vi "test-unscented-kalman-filter-0.vi"() -> (3 "All Tests Good":bool)   [LabVIEW 2019]
uses:
  <vilib>/Rock Robotics/WPI/ThirdParty/JAS_Junk/TrajLib/UNSCENTED_KALMAN_FILTER.ctl
  <vilib>/Analysis/Matrix/Datatypes/RealMatrix.ctl
  <vilib>/Rock Robotics/WPI/ThirdParty/JAS_Junk/TrajLib/MERWE_SCALED_SIGMA_PTS.ctl
  <vilib>/Rock Robotics/WPI/ThirdParty/JAS_Junk/TrajLib/CALLBACK_FUNC_TYPE.ctl
  <vilib>/Rock Robotics/WPI/ThirdParty/JAS_Junk/TrajLib/Rotation2d_CreateAngle.vi
  <vilib>/Rock Robotics/WPI/ThirdParty/JAS_Junk/TrajLib/Translation2d_Create.vi
  <vilib>/Rock Robotics/WPI/ThirdParty/JAS_Junk/TrajLib/Trajectory_Library.lvlib
  <vilib>/Analysis/Matrix/NI_Matrix.lvlib
panel:
  out "Error 7":bool
  out "JacobU":T1
  out "Y 2":T1
  out "out UnscentedKalmanFiilter 6":T2
  out "Error 6":bool
  out "out UnscentedKalmanFiilter 5":T2
  out "Error 5":bool
  out "out UnscentedKalmanFiilter 4":T2
  out "Error 4":errorcluster
  out "UnscentedKalmanFiilter 2":T2
  out "Y":T1
  out "out UnscentedKalmanFiilter 3":T2
  out "Error 3":bool
  out "out UnscentedKalmanFiilter 2":T2
  out "Error 2":bool
  out "out UnscentedKalmanFiilter":T2
  out "Error":errorcluster
  out "UnscentedKalmanFiilter":T2
  # "State Estimate <Statess,1>"
  # "<States, States>"
  # "<States, ?>"
  # "<Statess,  States>"
  # "<Outputs, Outputs>"
  # "<?, 1>"
  # "<?, 1>"
  # "State Estimate <Statess,1>"
  # "<States, States>"
  # "<States, ?>"
  # "<Statess,  States>"
  # "<Outputs, Outputs>"
  # "<?, 1>"
  # "<?, 1>"
  # "State Estimate <Statess,1>"
  # "<States, States>"
  # "<States, ?>"
  # "<Statess,  States>"
  # "<Outputs, Outputs>"
  # "<?, 1>"
  # "<?, 1>"
  # "State Estimate <Statess,1>"
  # "<States, States>"
  # "<States, ?>"
  # "<Statess,  States>"
  # "<Outputs, Outputs>"
  # "<?, 1>"
  # "<?, 1>"
  # "State Estimate <Statess,1>"
  # "<States, States>"
  # "<States, ?>"
  # "<Statess,  States>"
  # "<Outputs, Outputs>"
  # "<?, 1>"
  # "<?, 1>"
  # "State Estimate <Statess,1>"
  # "<States, States>"
  # "<States, ?>"
  # "<Statess,  States>"
  # "<Outputs, Outputs>"
  # "<?, 1>"
  # "<?, 1>"
  # "State Estimate <Statess,1>"
  # "<States, States>"
  # "<States, ?>"
  # "<Statess,  States>"
  # "<Outputs, Outputs>"
  # "<?, 1>"
  # "<?, 1>"
  # "State Estimate <Statess,1>"
  # "<States, States>"
  # "<States, ?>"
  # "<Statess,  States>"
  # "<Outputs, Outputs>"
  # "<?, 1>"
  # "<?, 1>"
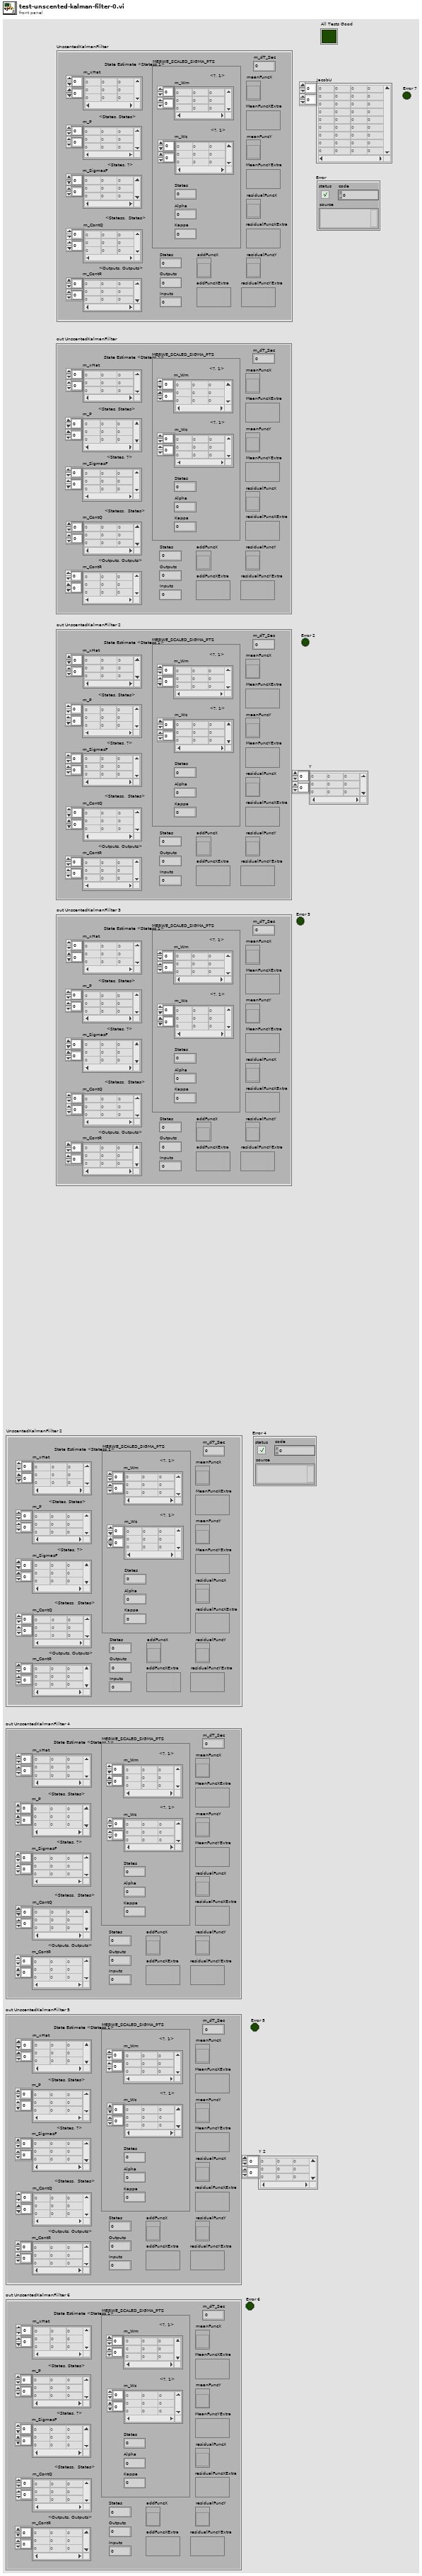
[diagram p1: front panel]
types:
  T1 = typedef "NI_Matrix.lvlib/RealMatrix.ctl" = dbl[][]
  T2 = typedef "Trajectory_Library.lvlib/UNSCENTED_KALMAN_FILTER.ctl" = cluster{"m_P":T1, "m_xHat":T1, "States":i32, "Outputs":i32, "m_ContR":T1, "m_ContQ":T1, "m_SigmasF":T1, "m_dT_Sec":dbl, "MERWE_SCALED_SIGMA_PTS":T3, "meanFuncX":T4, "meanFuncY":T4, "residualFuncX":T4, "residualFuncY":T4, "addFuncX":T4, "addFuncXExtra":variant, "residualFuncYExtra":variant, "residualFuncXExtra":variant, "MeanFuncYExtra":variant, "MeanFuncXExtra":variant, "Inputs":i32}
  T3 = typedef "Trajectory_Library.lvlib/MERWE_SCALED_SIGMA_PTS.ctl" = cluster{"m_Wm":T1, "States":i32, "Alpha":dbl, "m_Wc":T1, "Kappa":i32}
  T4 = typedef "Trajectory_Library.lvlib/CALLBACK_FUNC_TYPE.ctl" = refnum<vi>
  T5 = typedef "Trajectory_Library.lvlib/POSE2D.ctl" = cluster{"TRANSLATION":T6, "ROTATION":T7}
  T6 = typedef "Trajectory_Library.lvlib/TRANSLATION2D.ctl" = cluster{"X":dbl, "Y":dbl}
  T7 = typedef "Trajectory_Library.lvlib/ROTATION2D.ctl" = cluster{"VALUE":dbl, "COS":dbl, "SIN":dbl}
  T8 = typedef "Trajectory_Library.lvlib/TRAJ_CONFIG.ctl" = cluster{"MaxVelocity":dbl, "Max Acceleration":dbl, "StartVelocity":dbl, "End Velocity":dbl, "Reversed":bool, "DiffDrKineConstntDefined":bool, "CentAcellConstntDefined":bool, "DiffDrVoltConstntDefined":bool, "DIFF_DRIVE_KINE_CONSTRAINT":T9, "CENTRIPETAL_ACCEL_CONSTRAINT":T11, "SwerveDrKineConstntDefined":bool, "SWERVE_DRIVE_KINE_CONSTRAINT":T12, "DIFF_DRIVE_VOLTAGE_CONSTRAINT":T14, "MECANUM_DRIVE_KINE_CONSTRAINT":T16, "MecanumDrKineConstntDefined":bool}
  T9 = typedef "Trajectory_Library.lvlib/TRAJ_CONSTRAINT_DIIF_DRIVE_KINEMATICS.ctl" = cluster{"Max Speed (M/S)":dbl, "DIFF_DRIVE_KINEMATICS":T10, "Max Accel (M/S2)":dbl}
  T10 = typedef "Trajectory_Library.lvlib/DIFF_DRIVE_KINEMATICS.ctl" = cluster{"TrackWidth_Meters":dbl}
  T11 = typedef "Trajectory_Library.lvlib/TRAJ_CONSTRAINT_CENTRIPETAL_ACCEL.ctl" = cluster{"Max Cent Accel":dbl}
  T12 = typedef "Trajectory_Library.lvlib/TRAJ_CONSTRAINT_SWERVE_DRIVE_KINEMATICS.ctl" = cluster{"Max Speed (M/S)":dbl, "SwerveKinematics":T13}
  T13 = typedef "Trajectory_Library.lvlib/SWERVE_DRIVE_KINEMATICS.ctl" = cluster{"NumModules":i32, "InverseKinematics":T1, "ForwardKinematics":T1, "Modules":T6[], "PrevCoR":T6}
  T14 = typedef "Trajectory_Library.lvlib/TRAJ_CONSTRAINT_DIIF_DRIVE_VOLTAGE.ctl" = cluster{"Max Voltage":dbl, "DIFF_DRIVE_KINEMATICS":T10, "SIMPLE_MOTOR_FF":T15}
  T15 = typedef "Trajectory_Library.lvlib/SIMPLE_MOTOR_FF.ctl" = cluster{"Ks":dbl, "Kv":dbl, "Ka":dbl}
  T16 = typedef "Trajectory_Library.lvlib/TRAJ_CONSTRAINT_MECA_DRIVE_KINEMATICS.ctl" = cluster{"Max Speed (M/S)":dbl, "MECA_DRIVE_KINEMATICS":T17}
  T17 = typedef "Trajectory_Library.lvlib/MECA_DRIVE_KINEMATICS.ctl" = cluster{"FrontLeft":T6, "FrontRight":T6, "RearLeft":T6, "RearRight":T6, "InverseKinematics":T1, "ForwardKinematics":T1, "PrevCoR":T6}
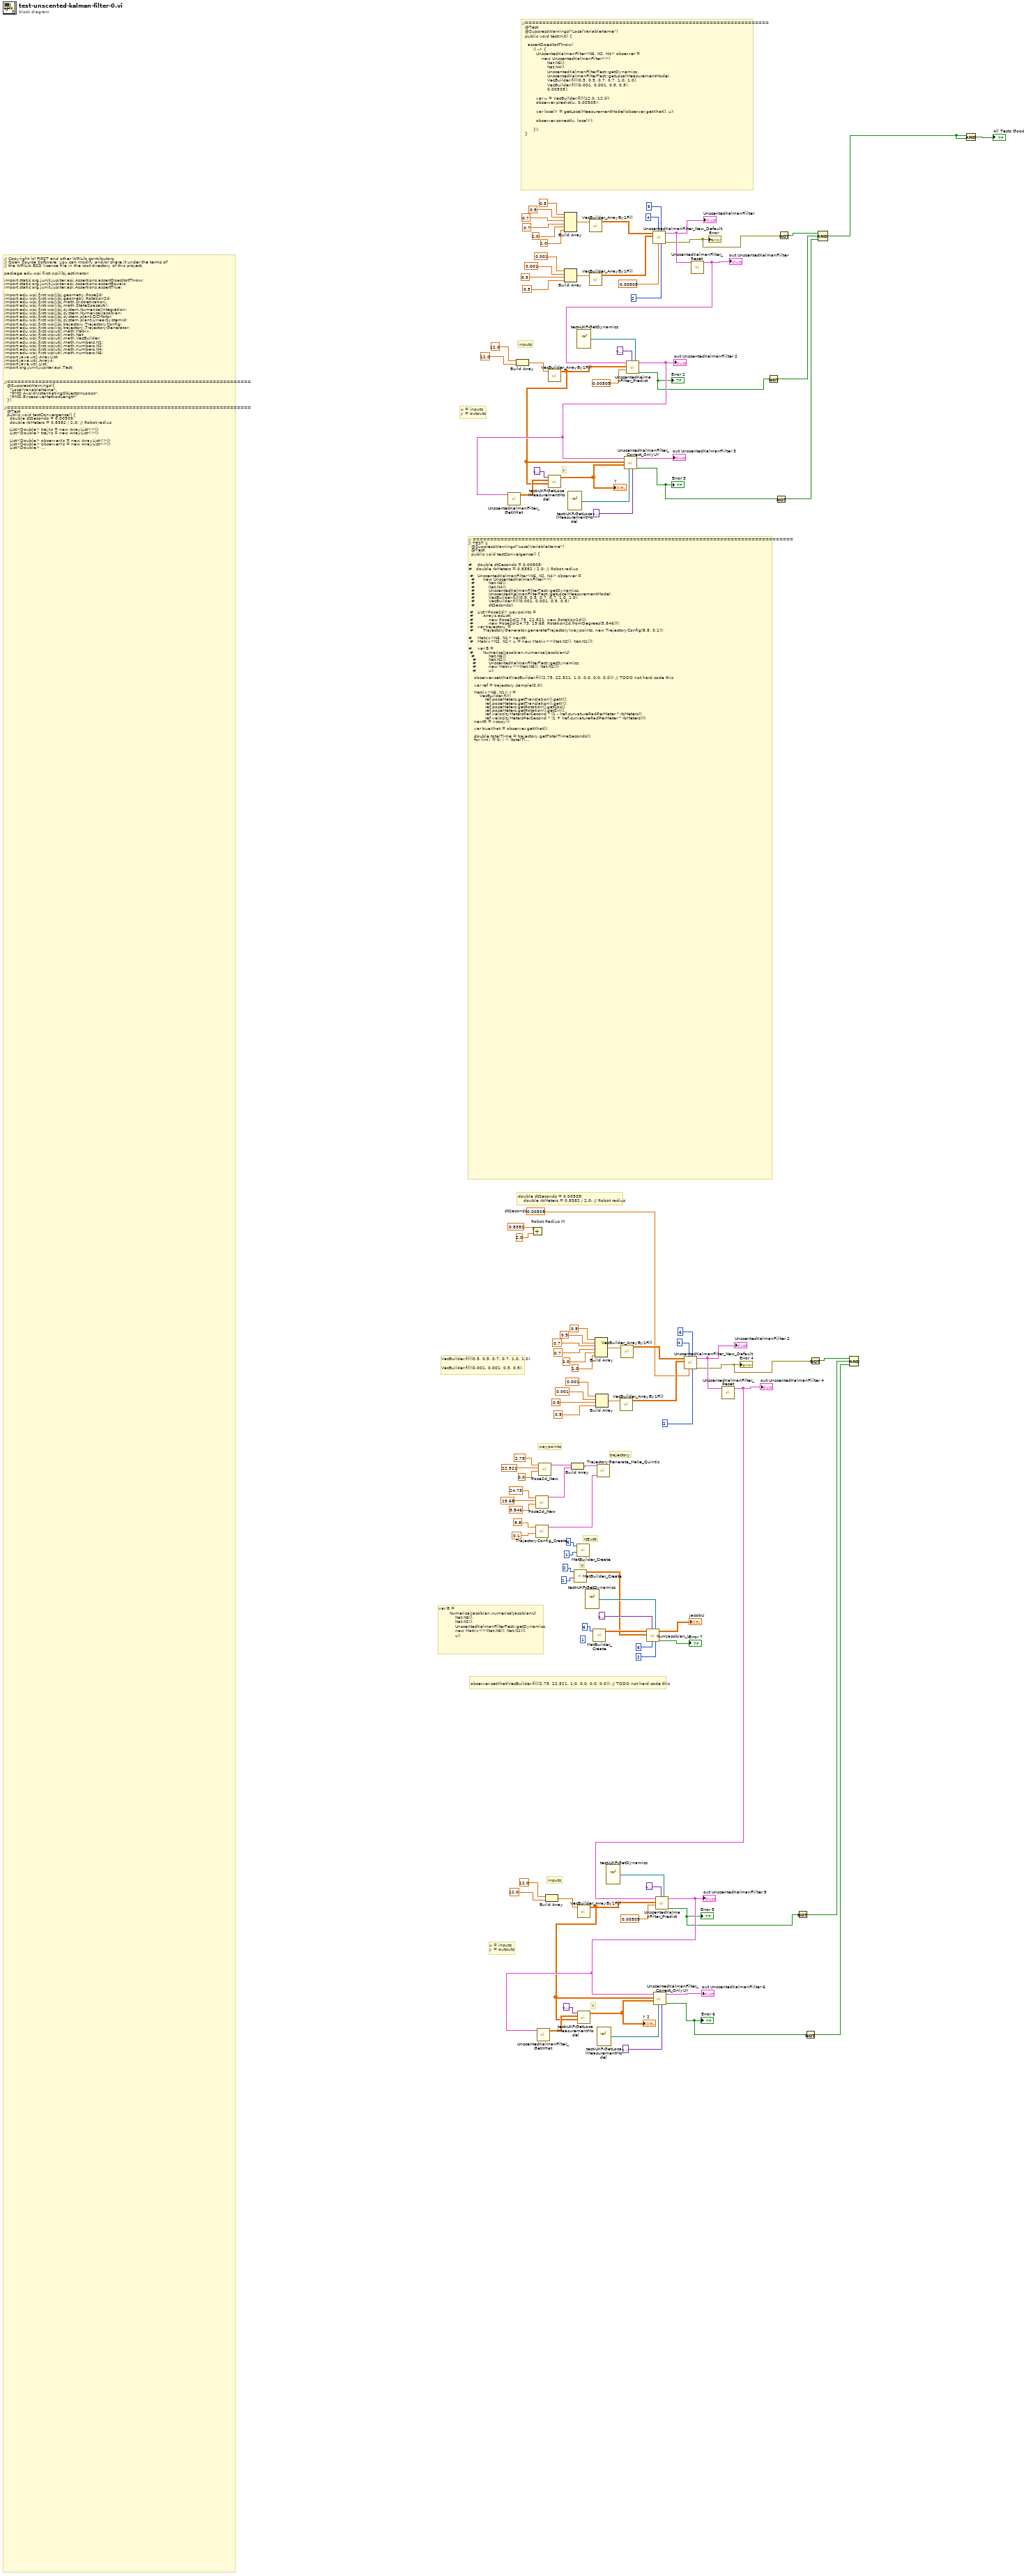
[diagram p0: block diagram]
diagram:
  (unwired) 1 ("Columns")
  w26 = 0.00505  # dtSeconds
  # "observer.setXhat(VecBuilder.fill(2.75, 22.521, 1.0, 0.0, 0.0, 0.0)); // TODO not hard code this"
  # "var B =\n        NumericalJacobian.numericalJacobianU(    \n            Nat.N6(),\n            Nat.N2(),\n            UnscentedKalmanFilterTest::getDynamics,\n            new Matrix<>(Nat.N6(), Nat.N1()),\n            u);"
  # "U"
  # "NExtR"
  # "trajectory"
  # "waypoints"
  # "VecBuilder.fill(0.5, 0.5, 0.7, 0.7, 1.0, 1.0),\n\nVecBuilder.fill(0.001, 0.001, 0.5, 0.5),"
  # "double dtSeconds = 0.00505;\n    double rbMeters = 0.8382 / 2.0; // Robot radius"
  # "u = inputs\ny = outputs"
  # "inputs"
  # "Y"
  # "// ============================================================================================\n// TEST 1\n  @SuppressWarnings(\"LocalVariableName\")\n  @Test\n  public void testConvergence() {\n\n\n#    double dtSeconds = 0.00505;\n#   double rbMeters = 0.8382 / 2.0; // Robot radius\n\n #   UnscentedKalmanFilter<N6, N2, N4> observer =\n  #      new UnscentedKalmanFilter<>(\n  #          Nat.N6(),\n  #          Nat.N4(),\n  #          UnscentedKalmanFilterTest::getDynamics,\n  #          UnscentedKalmanFilterTest::getLocalMeasurementModel,\n  #          VecBuilder.fill(0.5, 0.5, 0.7, 0.7, 1.0, 1.0),\n  #          VecBuilder.fill(0.001, 0.001, 0.5, 0.5),\n  #          dtSeconds);\n\n #   List<Pose2d> waypoints =\n #       Arrays.asList(\n #           new Pose2d(2.75, 22.521, new Rotation2d()),\n #           new Pose2d(24.73, 19.68, Rotation2d.fromDegrees(5.846)));\n #   var trajectory =\n #       TrajectoryGenerator.generateTrajectory(waypoints, new TrajectoryConfig(8.8, 0.1));\n\n#    Matrix<N6, N1> nextR;\n #   Matrix<N2, N1> u = new Matrix<>(Nat.N2(), Nat.N1());\n\n#    var B =\n #       NumericalJacobian.numericalJacobianU(  \n  #          Nat.N6(),\n   #         Nat.N2(),\n   #         UnscentedKalmanFilterTest::getDynamics,\n   #         new Matrix<>(Nat.N6(), Nat.N1()),\n   #         u);\n\n    observer.setXhat(VecBuilder.fill(2.75, 22.521, 1.0, 0.0, 0.0, 0.0)); // TODO not hard code this\n\n    var ref = trajectory.sample(0.0);\n\n    Matrix<N6, N1> r =\n        VecBuilder.fill(\n            ref.poseMeters.getTranslation().getX(),\n            ref.poseMeters.getTranslation().getY(),\n            ref.poseMeters.getRotation().getCos(),\n            ref.poseMeters.getRotation().getSin(),\n            ref.velocityMetersPerSecond * (1 - (ref.curvatureRadPerMeter * rbMeters)),\n            ref.velocityMetersPerSecond * (1 + (ref.curvatureRadPerMeter * rbMeters)));\n    nextR = r.copy();\n\n    var trueXhat = observer.getXhat();\n\n    double totalTime = trajectory.getTotalTimeSeconds();\n    for (int i = 0; i < (totalTime / dtSeconds); i++) {\n      ref = trajectory.sample(dtSeconds * i);\n      double vl = ref.velocityMetersPerSecond * (1 - (ref.curvatureRadPerMeter * rbMeters));\n      double vr = ref.velocityMetersPerSecond * (1 + (ref.curvatureRadPerMeter * rbMeters));\n\n      nextR.set(0, 0, ref.poseMeters.getTranslation().getX());\n      nextR.set(1, 0, ref.poseMeters.getTranslation().getY());\n      nextR.set(2, 0, ref.poseMeters.getRotation().getCos());\n      nextR.set(3, 0, ref.poseMeters.getRotation().getSin());\n      nextR.set(4, 0, vl);\n      nextR.set(5, 0, vr);\n\n      Matrix<N4, N1> localY = getLocalMeasurementModel(trueXhat, new Matrix<>(Nat.N2(), Nat.N1()));\n      var noiseStdDev = VecBuilder.fill(0.001, 0.001, 0.5, 0.5);\n\n      observer.correct(u, localY.plus(StateSpaceUtil.makeWhiteNoiseVector(noiseStdDev)));\n\n      var rdot = nextR.minus(r).div(dtSeconds);\n      u = new Matrix<>(B.solve(rdot.minus(getDynamics(r, new Matrix<>(Nat.N2(), Nat.N1())))));\n\n      r = nextR;\n      observer.predict(u, dtSeconds);\n      trueXhat =\n          NumericalIntegration.rk4(UnscentedKalmanFilterTest::getDynamics, trueXhat, u, dtSeconds);\n    }\n\n    var localY = getLocalMeasurementModel(trueXhat, u);\n    observer.correct(u, localY);\n\n    var globalY = getGlobalMeasurementModel(trueXhat, u);\n    var R = StateSpaceUtil.makeCostMatrix(VecBuilder.fill(0.01, 0.01, 0.0001, 0.0001, 0.5, 0.5));\n    observer.correct(\n        Nat.N6(),\n        u,\n        globalY,\n        UnscentedKalmanFilterTest::getGlobalMeasurementModel,\n        R,\n        (sigmas, weights) -> sigmas.times(Matrix.changeBoundsUnchecked(weights)),\n        Matrix::minus,\n        Matrix::minus,\n        Matrix::plus);\n\n    final var finalPosition = trajectory.sample(trajectory.getTotalTimeSeconds());\n\n    assertEquals(finalPosition.poseMeters.getTranslation().getX(), observer.getXhat(0), 0.25);\n    assertEquals(finalPosition.poseMeters.getTranslation().getY(), observer.getXhat(1), 0.25);\n    assertEquals(finalPosition.poseMeters.getRotation().getRadians(), observer.getXhat(2), 1.0);\n    assertEquals(0.0, observer.getXhat(3), 1.0);\n    assertEquals(0.0, observer.getXhat(4), 1.0);\n  }"
  # "u = inputs\ny = outputs"
  # "inputs"
  # "Y"
  # "//======================================================================\n  @Test\n  @SuppressWarnings(\"LocalVariableName\")\n  public void testInit() {\n\n    assertDoesNotThrow(\n        () -> {\n          UnscentedKalmanFilter<N6, N2, N4> observer =\n              new UnscentedKalmanFilter<>(\n                  Nat.N6(),\n                  Nat.N4(),\n                  UnscentedKalmanFilterTest::getDynamics,\n                  UnscentedKalmanFilterTest::getLocalMeasurementModel,\n                  VecBuilder.fill(0.5, 0.5, 0.7, 0.7, 1.0, 1.0),\n                  VecBuilder.fill(0.001, 0.001, 0.5, 0.5),\n                  0.00505);\n\n          var u = VecBuilder.fill(12.0, 12.0);\n          observer.predict(u, 0.00505);\n\n          var localY = getLocalMeasurementModel(observer.getXhat(), u);\n\n          observer.correct(u, localY);\n\n        });\n  }"
  # "// Copyright (c) FIRST and other WPILib contributors.\n// Open Source Software; you can modify and/or share it under the terms of\n// the WPILib BSD license file in the root directory of this project.\n\npackage edu.wpi.first.wpilibj.estimator;\n\nimport static org.junit.jupiter.api.Assertions.assertDoesNotThrow;\nimport static org.junit.jupiter.api.Assertions.assertEquals;\nimport static org.junit.jupiter.api.Assertions.assertTrue;\n\nimport edu.wpi.first.wpilibj.geometry.Pose2d;\nimport edu.wpi.first.wpilibj.geometry.Rotation2d;\nimport edu.wpi.first.wpilibj.math.Discretization;\nimport edu.wpi.first.wpilibj.math.StateSpaceUtil;\nimport edu.wpi.first.wpilibj.system.NumericalIntegration;\nimport edu.wpi.first.wpilibj.system.NumericalJacobian;\nimport edu.wpi.first.wpilibj.system.plant.DCMotor;\nimport edu.wpi.first.wpilibj.system.plant.LinearSystemId;\nimport edu.wpi.first.wpilibj.trajectory.TrajectoryConfig;\nimport edu.wpi.first.wpilibj.trajectory.TrajectoryGenerator;\nimport edu.wpi.first.wpiutil.math.Matrix;\nimport edu.wpi.first.wpiutil.math.Nat;\nimport edu.wpi.first.wpiutil.math.VecBuilder;\nimport edu.wpi.first.wpiutil.math.numbers.N1;\nimport edu.wpi.first.wpiutil.math.numbers.N2;\nimport edu.wpi.first.wpiutil.math.numbers.N4;\nimport edu.wpi.first.wpiutil.math.numbers.N6;\nimport java.util.ArrayList;\nimport java.util.Arrays;\nimport java.util.List;\nimport org.junit.jupiter.api.Test;\n\n\n\n//======================================================================\n  @SuppressWarnings({\n    \"LocalVariableName\",\n    \"PMD.AvoidInstantiatingObjectsInLoops\",\n    \"PMD.ExcessiveMethodLength\"\n  })\n\n//======================================================================\n  @Test\n  public void testConvergence() {\n    double dtSeconds = 0.00505;\n    double rbMeters = 0.8382 / 2.0; // Robot radius\n\n    List<Double> trajXs = new ArrayList<>();\n    List<Double> trajYs = new ArrayList<>();\n\n    List<Double> observerXs = new ArrayList<>();\n    List<Double> observerYs = new ArrayList<>();\n    List<Double> observerC = new ArrayList<>();\n    List<Double> observerS = new ArrayList<>();\n    List<Double> observervl = new ArrayList<>();\n    List<Double> observervr = new ArrayList<>();\n\n    List<Double> inputVl = new ArrayList<>();\n    List<Double> inputVr = new ArrayList<>();\n\n    List<Double> timeData = new ArrayList<>();\n    List<Matrix<?, ?>> rdots = new ArrayList<>();\n\n    UnscentedKalmanFilter<N6, N2, N4> observer =\n        new UnscentedKalmanFilter<>(\n            Nat.N6(),\n            Nat.N4(),\n            UnscentedKalmanFilterTest::getDynamics,\n            UnscentedKalmanFilterTest::getLocalMeasurementModel,\n            VecBuilder.fill(0.5, 0.5, 0.7, 0.7, 1.0, 1.0),\n            VecBuilder.fill(0.001, 0.001, 0.5, 0.5),\n            dtSeconds);\n\n    List<Pose2d> waypoints =\n        Arrays.asList(\n            new Pose2d(2.75, 22.521, new Rotation2d()),\n            new Pose2d(24.73, 19.68, Rotation2d.fromDegrees(5.846)));\n    var trajectory =\n        TrajectoryGenerator.generateTrajectory(waypoints, new TrajectoryConfig(8.8, 0.1));\n\n    Matrix<N6, N1> nextR;\n    Matrix<N2, N1> u = new Matrix<>(Nat.N2(), Nat.N1());\n\n    var B =\n        NumericalJacobian.numericalJacobianU(\n            Nat.N6(),\n            Nat.N2(),\n            UnscentedKalmanFilterTest::getDynamics,\n            new Matrix<>(Nat.N6(), Nat.N1()),\n            u);\n\n    observer.setXhat(VecBuilder.fill(2.75, 22.521, 1.0, 0.0, 0.0, 0.0)); // TODO not hard code this\n\n    var ref = trajectory.sample(0.0);\n\n    Matrix<N6, N1> r =\n        VecBuilder.fill(\n            ref.poseMeters.getTranslation().getX(),\n            ref.poseMeters.getTranslation().getY(),\n            ref.poseMeters.getRotation().getCos(),\n            ref.poseMeters.getRotation().getSin(),\n            ref.velocityMetersPerSecond * (1 - (ref.curvatureRadPerMeter * rbMeters)),\n            ref.velocityMetersPerSecond * (1 + (ref.curvatureRadPerMeter * rbMeters)));\n    nextR = r.copy();\n\n    var trueXhat = observer.getXhat();\n\n    double totalTime = trajectory.getTotalTimeSeconds();\n    for (int i = 0; i < (totalTime / dtSeconds); i++) {\n\n      ref = trajectory.sample(dtSeconds * i);\n      double vl = ref.velocityMetersPerSecond * (1 - (ref.curvatureRadPerMeter * rbMeters));\n      double vr = ref.velocityMetersPerSecond * (1 + (ref.curvatureRadPerMeter * rbMeters));\n\n      nextR.set(0, 0, ref.poseMeters.getTranslation().getX());\n      nextR.set(1, 0, ref.poseMeters.getTranslation().getY());\n      nextR.set(2, 0, ref.poseMeters.getRotation().getCos());\n      nextR.set(3, 0, ref.poseMeters.getRotation().getSin());\n      nextR.set(4, 0, vl);\n      nextR.set(5, 0, vr);\n\n      Matrix<N4, N1> localY = getLocalMeasurementModel(trueXhat, new Matrix<>(Nat.N2(), Nat.N1()));\n      var noiseStdDev = VecBuilder.fill(0.001, 0.001, 0.5, 0.5);\n\n      observer.correct(u, localY.plus(StateSpaceUtil.makeWhiteNoiseVector(noiseStdDev)));\n\n      var rdot = nextR.minus(r).div(dtSeconds);\n      u = new Matrix<>(B.solve(rdot.minus(getDynamics(r, new Matrix<>(Nat.N2(), Nat.N1())))));\n\n      rdots.add(rdot);\n\n      trajXs.add(ref.poseMeters.getTranslation().getX());\n      trajYs.add(ref.poseMeters.getTranslation().getY());\n\n      observerXs.add(observer.getXhat().get(0, 0));\n      observerYs.add(observer.getXhat().get(1, 0));\n\n      observerC.add(observer.getXhat(2));\n      observerS.add(observer.getXhat(3));\n\n      observervl.add(observer.getXhat(4));\n      observervr.add(observer.getXhat(5));\n\n      inputVl.add(u.get(0, 0));\n      inputVr.add(u.get(1, 0));\n\n      timeData.add(i * dtSeconds);\n\n      r = nextR;\n      observer.predict(u, dtSeconds);\n      trueXhat =\n          NumericalIntegration.rk4(UnscentedKalmanFilterTest::getDynamics, trueXhat, u, dtSeconds);\n    }\n\n    var localY = getLocalMeasurementModel(trueXhat, u);\n    observer.correct(u, localY);\n\n    var globalY = getGlobalMeasurementModel(trueXhat, u);\n    var R = StateSpaceUtil.makeCostMatrix(VecBuilder.fill(0.01, 0.01, 0.0001, 0.0001, 0.5, 0.5));\n    observer.correct(\n        Nat.N6(),\n        u,\n        globalY,\n        UnscentedKalmanFilterTest::getGlobalMeasurementModel,\n        R,\n        (sigmas, weights) -> sigmas.times(Matrix.changeBoundsUnchecked(weights)),\n        Matrix::minus,\n        Matrix::minus,\n        Matrix::plus);\n\n    final var finalPosition = trajectory.sample(trajectory.getTotalTimeSeconds());\n\n    //     var chartBuilder = new XYChartBuilder();\n    //     chartBuilder.title = \"The Magic of Sensor Fusion, now with a \"\n    //           + observer.getClass().getSimpleName();\n    //     var xyPosChart = chartBuilder.build();\n\n    //     xyPosChart.setXAxisTitle(\"X pos, meters\");\n    //     xyPosChart.setYAxisTitle(\"Y pos, meters\");\n    //     xyPosChart.addSeries(\"Trajectory\", trajXs, trajYs);\n    //     xyPosChart.addSeries(\"xHat\", observerXs, observerYs);\n\n    //     var stateChart = new XYChartBuilder()\n    //           .title(\"States (x-hat)\").build();\n    //     stateChart.addSeries(\"Cos\", timeData, observerC);\n    //     stateChart.addSeries(\"Sin\", timeData, observerS);\n    //     stateChart.addSeries(\"vl, m/s\", timeData, observervl);\n    //     stateChart.addSeries(\"vr, m/s\", timeData, observervr);\n\n    //     var inputChart = new XYChartBuilder().title(\"Inputs\").build();\n    //     inputChart.addSeries(\"Left voltage\", timeData, inputVl);\n    //     inputChart.addSeries(\"Right voltage\", timeData, inputVr);\n\n    //     var rdotChart = new XYChartBuilder().title(\"Rdot\").build();\n    //     rdotChart.addSeries(\"xdot, or vx\", timeData, rdots.stream().map(it -> it.get(0, 0))\n    //           .collect(Collectors.toList()));\n    //     rdotChart.addSeries(\"ydot, or vy\", timeData, rdots.stream().map(it -> it.get(1, 0))\n    //           .collect(Collectors.toList()));\n    //     rdotChart.addSeries(\"cos dot\", timeData, rdots.stream().map(it -> it.get(2, 0))\n    //           .collect(Collectors.toList()));\n    //     rdotChart.addSeries(\"sin dot\", timeData, rdots.stream().map(it -> it.get(3, 0))\n    //           .collect(Collectors.toList()));\n    //     rdotChart.addSeries(\"vl dot, or al\", timeData, rdots.stream().map(it -> it.get(4, 0))\n    //           .collect(Collectors.toList()));\n    //     rdotChart.addSeries(\"vr dot, or ar\", timeData, rdots.stream().map(it -> it.get(5, 0))\n    //           .collect(Collectors.toList()));\n\n    //     List<XYChart> charts = new ArrayList<>();\n    //     charts.add(xyPosChart);\n    //     charts.add(stateChart);\n    //     charts.add(inputChart);\n    //     charts.add(rdotChart);\n    //     new SwingWrapper<>(charts).displayChartMatrix();\n    //     try {\n    //       Thread.sleep(1000000000);\n    //     } catch (InterruptedException ex) {\n    //       ex.printStackTrace();\n    //     }\n\n    assertEquals(finalPosition.poseMeters.getTranslation().getX(), observer.getXhat(0), 0.25);\n    assertEquals(finalPosition.poseMeters.getTranslation().getY(), observer.getXhat(1), 0.25);\n    assertEquals(finalPosition.poseMeters.getRotation().getRadians(), observer.getXhat(2), 1.0);\n    assertEquals(0.0, observer.getXhat(3), 1.0);\n    assertEquals(0.0, observer.getXhat(4), 1.0);\n  }\n\n//======================================================================\n  @Test\n  @SuppressWarnings({\"LocalVariableName\", \"ParameterName\", \"PMD.AvoidInstantiatingObjectsInLoops\"})\n  public void testLinearUKF() {\n    var dt = 0.020;\n    var plant = LinearSystemId.identifyVelocitySystem(0.02, 0.006);\n    var observer =\n        new UnscentedKalmanFilter<>(\n            Nat.N1(),\n            Nat.N1(),\n            (x, u) -> plant.getA().times(x).plus(plant.getB().times(u)),\n            plant::calculateY,\n            VecBuilder.fill(0.05),\n            VecBuilder.fill(1.0),\n            dt);\n\n    var time = new ArrayList<Double>();\n    var refData = new ArrayList<Double>();\n    var xhat = new ArrayList<Double>();\n    var udata = new ArrayList<Double>();\n    var xdotData = new ArrayList<Double>();\n\n    var discABPair = Discretization.discretizeAB(plant.getA(), plant.getB(), dt);\n    var discA = discABPair.getFirst();\n    var discB = discABPair.getSecond();\n\n    Matrix<N1, N1> ref = VecBuilder.fill(100);\n    Matrix<N1, N1> u = VecBuilder.fill(0);\n\n    Matrix<N1, N1> xdot;\n    for (int i = 0; i < (2.0 / dt); i++) {\n      observer.predict(u, dt);\n\n      u = discB.solve(ref.minus(discA.times(ref)));\n\n      xdot = plant.getA().times(observer.getXhat()).plus(plant.getB().times(u));\n\n      time.add(i * dt);\n      refData.add(ref.get(0, 0));\n      xhat.add(observer.getXhat(0));\n      udata.add(u.get(0, 0));\n      xdotData.add(xdot.get(0, 0));\n    }\n\n    //    var chartBuilder = new XYChartBuilder();\n    //    chartBuilder.title = \"The Magic of Sensor Fusion\";\n    //    var chart = chartBuilder.build();\n\n    //    chart.addSeries(\"Ref\", time, refData);\n    //    chart.addSeries(\"xHat\", time, xhat);\n    //    chart.addSeries(\"input\", time, udata);\n    ////    chart.addSeries(\"xdot\", time, xdotData);\n\n    //    new SwingWrapper<>(chart).displayChart();\n    //    try {\n    //      Thread.sleep(1000000000);\n    //    } catch (InterruptedException e) {\n    //    }\n\n    assertEquals(ref.get(0, 0), observer.getXhat(0), 5);\n  }\n\n//======================================================================\n  @Test\n  public void testUnscentedTransform() {\n    // From FilterPy\n    var ret =\n        UnscentedKalmanFilter.unscentedTransform(\n            Nat.N4(),\n            Nat.N4(),\n            Matrix.mat(Nat.N4(), Nat.N9())\n                .fill(\n                    -0.9,\n                    -0.822540333075852,\n                    -0.8922540333075852,\n                    -0.9,\n                    -0.9,\n                    -0.9774596669241481,\n                    -0.9077459666924148,\n                    -0.9,\n                    -0.9,\n                    1.0,\n                    1.0,\n                    1.077459666924148,\n                    1.0,\n                    1.0,\n                    1.0,\n                    0.9225403330758519,\n                    1.0,\n                    1.0,\n                    -0.9,\n                    -0.9,\n                    -0.9,\n                    -0.822540333075852,\n                    -0.8922540333075852,\n                    -0.9,\n                    -0.9,\n                    -0.9774596669241481,\n                    -0.9077459666924148,\n                    1.0,\n                    1.0,\n                    1.0,\n                    1.0,\n                    1.077459666924148,\n                    1.0,\n                    1.0,\n                    1.0,\n                    0.9225403330758519),\n            VecBuilder.fill(\n                -132.33333333,\n                16.66666667,\n                16.66666667,\n                16.66666667,\n                16.66666667,\n                16.66666667,\n                16.66666667,\n                16.66666667,\n                16.66666667),\n            VecBuilder.fill(\n                -129.34333333,\n                16.66666667,\n                16.66666667,\n                16.66666667,\n                16.66666667,\n                16.66666667,\n                16.66666667,\n                16.66666667,\n                16.66666667),\n            (sigmas, weights) -> sigmas.times(Matrix.changeBoundsUnchecked(weights)),\n            Matrix::minus);\n\n    assertTrue(VecBuilder.fill(-0.9, 1, -0.9, 1).isEqual(ret.getFirst(), 1E-5));\n\n    assertTrue(\n        Matrix.mat(Nat.N4(), Nat.N4())\n            .fill(\n                2.02000002e-01,\n                2.00000500e-02,\n                -2.69044710e-29,\n                -4.59511477e-29,\n                2.00000500e-02,\n                2.00001000e-01,\n                -2.98781068e-29,\n                -5.12759588e-29,\n                -2.73372625e-29,\n                -3.09882635e-29,\n                2.02000002e-01,\n                2.00000500e-02,\n                -4.67065917e-29,\n                -5.10705197e-29,\n                2.00000500e-02,\n                2.00001000e-01)\n            .isEqual(ret.getSecond(), 1E-5));\n  }\n}"
  n1 = Build Array(12.0 ("element"), 12.0 ("element")) -> (w87:dbl[])
  n2 = Divide "Robot Radius M"(x=0.8382, y=2.0) -> ()  [unwired: 1 out]
  n3 = call <vilib>:"Pose2d_New.vi"("Heading"=5.846, "Y"=19.68, "X"=24.73) -> ("out POSe"=w18:T5)  [unwired: 8 in]
  n4 = call <vilib>:"TrajectoryConfig_Create.vi"("MaxAcceleration"=0.1, "MaxVelocity"=8.8) -> ("TRAJECTORY_CONFIG"=w14:T8)  [unwired: 9 in]
  n5 = call <vilib>:"Pose2d_New.vi"("Heading"=0.0, "Y"=22.521, "X"=2.75) -> ("out POSe"=w19:T5)  [unwired: 8 in]
  n6 = Build Array(12.0 ("element"), 12.0 ("element")) -> (w46:dbl[])
  n7 = call <vilib>:"VecBuilder_ArrayBy1Fill.vi"("R Array"=w87) -> ("Output Vector"=w77:T1)  [unwired: 10 in]
  n8 = Build Array(0.5 ("element"), 0.5 ("element"), 0.7 ("element"), 0.7 ("element"), 1.0 ("element"), 1.0 ("element")) -> (w107:dbl[])
  n9 = Build Array(0.001 ("element"), 0.001 ("element"), 0.5 ("element"), 0.5 ("element")) -> (w96:dbl[])
  n10 = vi-ref "test-UKF-GetLocalMeasurementModel.vi"() -> (w82:refnum<vi>)
  n11 = Build Array(w19, w18) -> (w15:T5[])
  n12 = call <vilib>:"MatBuilder_Create.vi"("Columns"=1, "Rows"=2) -> ("output matrix"=w1:T1)  [unwired: 9 in]
  n13 = vi-ref "test-UKF-GetDynamics.vi"() -> (w84:refnum<vi>)
  n14 = call <vilib>:"MatBuilder_Create.vi"("Columns"=1, "Rows"=6) -> ()  [unwired: 9 in, 1 out]
  n15 = call <vilib>:"VecBuilder_ArrayBy1Fill.vi"("R Array"=w46) -> ("Output Vector"=w36:T1)  [unwired: 10 in]
  n16 = vi-ref "test-UKF-GetDynamics.vi"() -> (w9:refnum<vi>)
  n17 = call <vilib>:"VecBuilder_ArrayBy1Fill.vi"("R Array"=w96) -> ("Output Vector"=w95:T1)  [unwired: 10 in]
  n18 = call <vilib>:"VecBuilder_ArrayBy1Fill.vi"("R Array"=w107) -> ("Output Vector"=w94:T1)  [unwired: 10 in]
  n19 = call <vilib>:"MatBuilder_Create.vi"("Rows"=6) -> ("output matrix"=w2:T1)  [unwired: 10 in]
  n20 = Build Array(0.5 ("element"), 0.5 ("element"), 0.7 ("element"), 0.7 ("element"), 1.0 ("element"), 1.0 ("element")) -> (w65:dbl[])
  n21 = Build Array(0.001 ("element"), 0.001 ("element"), 0.5 ("element"), 0.5 ("element")) -> (w54:dbl[])
  n22 = call <vilib>:"TrajectoryGenerate_Make_Quintic.vi"("traj_config"=w14, "waypointPOSE"=w15) -> ()  [unwired: 8 in, 2 out]
  n23 = vi-ref "test-UKF-GetLocalMeasurementModel.vi"() -> (w41:refnum<vi>)
  n24 = vi-ref "test-UKF-GetDynamics.vi"() -> (w43:refnum<vi>)
  n25 = call <vilib>:"VecBuilder_ArrayBy1Fill.vi"("R Array"=w54) -> ("Output Vector"=w53:T1)  [unwired: 10 in]
  n26 = call <vilib>:"VecBuilder_ArrayBy1Fill.vi"("R Array"=w65) -> ("Output Vector"=w52:T1)  [unwired: 10 in]
  n27 = call <vilib>:"NumJacobian_U.vi"("Inputs"=2, "F_FUNC"=w9, "Rows"=6, "ExtraPassedData"=variant ("F_Func_ExtraData"), "U"=w1, "X"=w2) -> ("Error"=→"Error 7":bool, "Result"=→"JacobU":T1)  [unwired: 4 in]
  n28 = call <vilib>:"UnscentedKalmanFilter_New_Default.vi"("Inputs"=2, "States"=6, "dt_Seconds"=0.00505, "Outputs"=4, "MeasurementStdDevs"=w95, "StateStdDevs"=w94) -> ("Error"=w75:errorcluster, "UnscentedKalmanFiilter"=w91:T2)  [unwired: 4 in]
  "UnscentedKalmanFiilter" <- w91
  "Error" <- w75
  n29 = call <vilib>:"UnscentedKalmanFilter_New_Default.vi"("Inputs"=2, "States"=6, "dt_Seconds"=w26, "Outputs"=4, "MeasurementStdDevs"=w53, "StateStdDevs"=w52) -> ("Error"=w34:errorcluster, "UnscentedKalmanFiilter"=w50:T2)  [unwired: 4 in]
  "UnscentedKalmanFiilter 2" <- w50
  "Error 4" <- w34
  n30 = call <vilib>:"UnscentedKalmanFilter_Reset.vi"("in UnscentedKalmanFiilter"=w91) -> ("out UnscentedKalmanFiilter"=w90:T2)  [unwired: 10 in]
  "out UnscentedKalmanFiilter" <- w90
  n31 = call <vilib>:"UnscentedKalmanFilter_Predict.vi"("f_Func"=w84, "F_Func_ExtraData"=variant, "dT_Seconds"=0.00505, "U"=w77, "in UnscentedKalmanFiilter"=w90) -> ("Error"=w73:bool, "out UnscentedKalmanFiilter"=w80:T2)  [unwired: 5 in]
  "Error 2" <- w73
  "out UnscentedKalmanFiilter 2" <- w80
  n32 = call <vilib>:"UnscentedKalmanFilter_GetXHat.vi"("in UnscentedKalmanFiilter"=w80) -> ("xHat"=w78:T1)  [unwired: 10 in]
  n33 = call "test-UKF-GetLocalMeasurementModel.vi"("U"=w77, "X"=w78, "Variant"=variant) -> ("Return"=w76:T1)  [unwired: 7 in, 1 out]
  "Y" <- w76
  n34 = call <vilib>:"UnscentedKalmanFilter_Correct_OnlyUY.vi"("H_ExtraData"=variant ("F_Func_ExtraData"), "H_Func"=w82, "Y"=w76, "U"=w77, "in UnscentedKalmanFiilter"=w80) -> ("Error"=w74:bool, "out UnscentedKalmanFiilter"=→"out UnscentedKalmanFiilter 3":T2)  [unwired: 5 in]
  "Error 3" <- w74
  n35 = call <vilib>:"UnscentedKalmanFilter_Reset.vi"("in UnscentedKalmanFiilter"=w50) -> ("out UnscentedKalmanFiilter"=w49:T2)  [unwired: 10 in]
  "out UnscentedKalmanFiilter 4" <- w49
  n36 = call <vilib>:"UnscentedKalmanFilter_Predict.vi"("f_Func"=w43, "F_Func_ExtraData"=variant, "dT_Seconds"=0.00505, "U"=w36, "in UnscentedKalmanFiilter"=w49) -> ("Error"=w32:bool, "out UnscentedKalmanFiilter"=w39:T2)  [unwired: 5 in]
  "Error 5" <- w32
  "out UnscentedKalmanFiilter 5" <- w39
  n37 = call <vilib>:"UnscentedKalmanFilter_GetXHat.vi"("in UnscentedKalmanFiilter"=w39) -> ("xHat"=w37:T1)  [unwired: 10 in]
  n38 = call "test-UKF-GetLocalMeasurementModel.vi"("U"=w36, "X"=w37, "Variant"=variant) -> ("Return"=w35:T1)  [unwired: 7 in, 1 out]
  "Y 2" <- w35
  n39 = call <vilib>:"UnscentedKalmanFilter_Correct_OnlyUY.vi"("H_ExtraData"=variant ("F_Func_ExtraData"), "H_Func"=w41, "Y"=w35, "U"=w36, "in UnscentedKalmanFiilter"=w39) -> ("Error"=w33:bool, "out UnscentedKalmanFiilter"=→"out UnscentedKalmanFiilter 6":T2)  [unwired: 5 in]
  "Error 6" <- w33
  n40 = Not(x=w73) -> (.not. x?=w71:bool)
  n41 = Not(x=w74) -> (.not. x?=w70:bool)
  n42 = Not(x=w75) -> (.not. x?=w72:bool)
  n43 = Not(x=w32) -> (.not. x?=w30:bool)
  n44 = Not(x=w33) -> (.not. x?=w29:bool)
  n45 = Not(x=w34) -> (.not. x?=w31:bool)
  n46 = Compound Arithmetic op=AND(w72, w71, w70) -> (w69:bool)
  n47 = Compound Arithmetic op=AND(w31, w30, w29) -> ()  [unwired: 1 out]
  n48 = Compound Arithmetic op=AND(w69, w69) -> (→"All Tests Good":bool)
